vi "Oxford Read Channel.vi"(8 "error in (no error)":errorcluster, 10 "Channel #":i32=1, 11 "VISA resource name":refnum<visa-resource-name>) -> (0 "error out":errorcluster, 1 "read buffer":string, 2 "Data":dbl, 3 "VISA resource name out":refnum<visa-resource-name>)   [LabVIEW 2015]
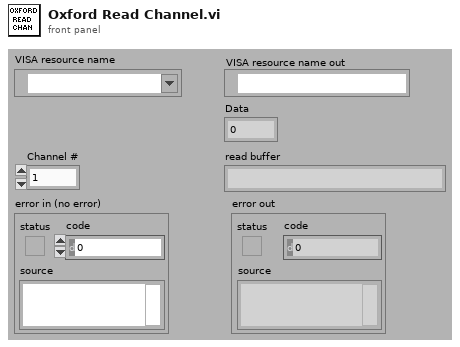
[diagram p1: front panel]
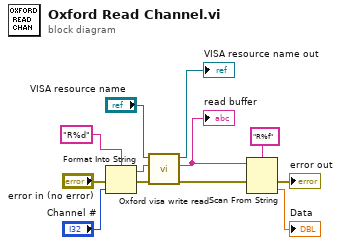
[diagram p0: block diagram]
diagram:
  n1 = Format Into String(format string="R%d" ("write buffer"), error in="error in (no error)", "Channel #") -> (resulting string=w6:string, error out=w9:errorcluster)  [unwired: 1 in]
  n2 = call "Oxford visa write read.vi"("error in (no error)"=w9, "write buffer"=w6, "VISA resource name"="VISA resource name") -> ("error out"=w5:errorcluster, "read buffer"=w1:string, "VISA resource name out"=→"VISA resource name out":refnum<visa-resource-name>)  [unwired: 6 in]
  "read buffer" <- w1
  n3 = Scan From String(format string="R%f", input string=w1, error in=w5) -> (error out=→"error out":errorcluster, output 1=→"Data":dbl)  [unwired: 2 in, 2 out]
